vi "RT FIFO Read AB.vi"(8 "error in":errorcluster, 10 "Elements to Read":u32=12000, 11 "FPGA VI Reference In":refnum<k20>) -> (0 "error out":errorcluster, 1 "FPGA VI Reference Out":refnum<k20>, 2 "to RT - elements \nremaining":u32=4095, 3 "data":i16[][](array[numeric]))   [LabVIEW 2018]
uses:
  <vilib>/Utility/error.llb/Error Cluster From Error Code.vi
  <vilib>/rvi/errors/niLvFpgaAdjustHostInterfaceError.vi
  <vilib>/rvi/interface/nirviMethod/nirviMethod.xnode
  <vilib>/FPGAPlugInAG/Dynamic/niLvFpga_ReadFifo_Dynamic.vi
  <vilib>/rvi/errors/niLvFpgaMergeErrorWithErrorCode.vi
  <vilib>/FPGAPlugInAG/Dynamic/niLvFpga_StartFifo_Dynamic.vi
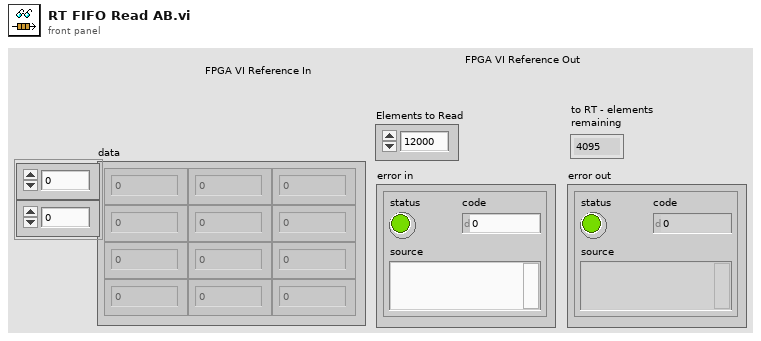
[diagram p1: front panel]
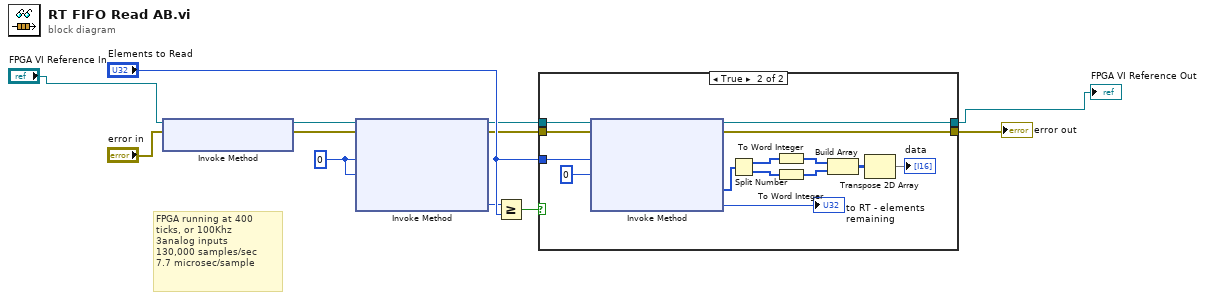
[diagram p0: block diagram]
diagram:
  w6 = u32 0 ("Number of Elements")
  # "FPGA running at 400 ticks, or 100Khz\n3analog inputs\n130,000 samples/sec\n7.7 microsec/sample"
  n1 = xnode "Invoke Method"("FPGA VI Reference In"="FPGA VI Reference In", "error in"="error in") -> ("FPGA VI Reference Out"=w12:refnum<k20>, "error out"=w11:errorcluster)
  n2 = xnode "Invoke Method"("FPGA VI Reference In"=w12, "error in"=w11, "Number of Elements"=w6, "Timeout (ms)"=w6) -> ("FPGA VI Reference Out"=w3:refnum<k20>, "error out"=w4:errorcluster, "Elements Remaining"=w5:u32)  [unwired: 1 out]
  n3 = Greater Or Equal?(x=w5, y="Elements to Read") -> (x >= y?=w7:bool)
  n4 = case shown="True" w7 {
    tunnel: "Elements to Read" -> [_ w27]
    tunnel: [w14 w26] -> w9
    tunnel: w4 -> [w14 w21]
    tunnel: w3 -> [w13 w20]
    tunnel: [w13 w19] -> w2
    frame False {
    }
    frame True {
      n5 = xnode "Invoke Method"("FPGA VI Reference In"=w20, "error in"=w21, "Number of Elements"=w27, "Timeout (ms)"=0) -> ("FPGA VI Reference Out"=w19:refnum<k20>, "error out"=w26:errorcluster, "Data"=w24:u32[], "Elements Remaining"=→"to RT - elements \nremaining":u32)
      n6 = Split Number(x=w24) -> (hi(x)=w17:u16[], lo(x)=w16:u16[])
      n7 = To Word Integer(number=w17) -> (16bit integer=w15:i16[])
      n8 = To Word Integer(number=w16) -> (16bit integer=w18:i16[])
      n9 = Build Array(w15, w18) -> (w25:i16[][])
      n10 = Transpose 2D Array(2D array=w25) -> (transposed array=→"data":i16[][])
    }
  }
  "error out" <- w9
  "FPGA VI Reference Out" <- w2
